vi "EndRoutine.vi"(9 "End?":bool, 10 "Ended Safe?":bool, 11 "End Time":timestamp) -> (3 "Stop?":bool)   [LabVIEW 2017]
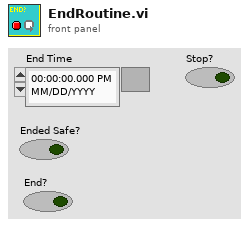
[diagram p1: front panel]
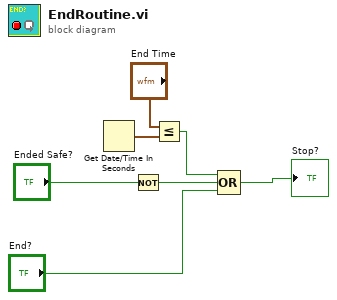
[diagram p0: block diagram]
diagram:
  n1 = Get Date/Time In Seconds() -> (seconds since 1Jan1904=w3:timestamp)
  n2 = Not(x="Ended Safe?") -> (.not. x?=w7:bool)
  n3 = Less Or Equal?(x="End Time", y=w3) -> (x <= y?=w5:bool)
  n4 = Compound Arithmetic op=OR(w5, w7, "End?") -> (→"Stop?":bool)
